vi "Adam_server_messages.vi"(1 "Filename":path) -> ()   [LabVIEW 2015]
panel:
  out "String":string
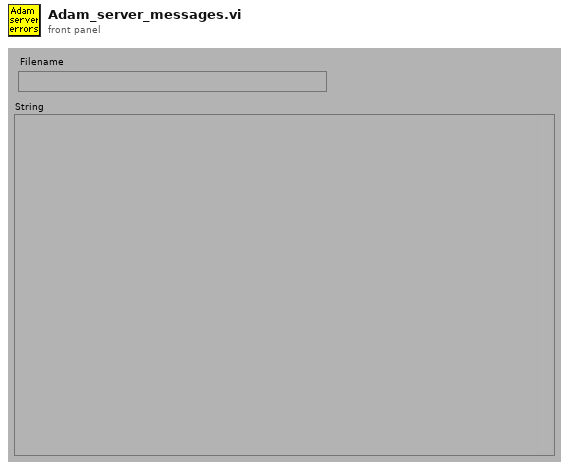
[diagram p1: front panel]
types:
  T1 = typedef "Ch_description_ADAM.ctl" = cluster{"Ch Name":string, "Type":T2, "Function":T3, "Ch State":T4, "Calibration type":T5, "A":dbl, "B":dbl, "C":dbl, "D":dbl, "Comments":string, "Address":T6, "String":string, "Duty":u16}
  T2 = typedef "Module_type_ADAM.ctl" = string
  T3 = typedef "Function_ADAM.ctl" = enum16{"Analogue Input", "Digital Input", "Event counter", "Event rate", "Analogue Output", "Digital Output", "Relay Output"}
  T4 = typedef "Channel_State.ctl" = enum16{"On", "Off", "Always On", "Always Off"}
  T5 = typedef "Calib_type_ADAM.ctl" = enum16{"Raw", "Bx + A", "Cx^2 + Bx + A", "Dx^3 + Cx^2 + Bx + A", "In Band", "Hi-Tec Q", "Hi-Tec M_dot", "Text"}
  T6 = typedef "Address.ctl" = cluster{"Main":i32, "Ch.":i32, "Sub":i32, "Port Name":string}
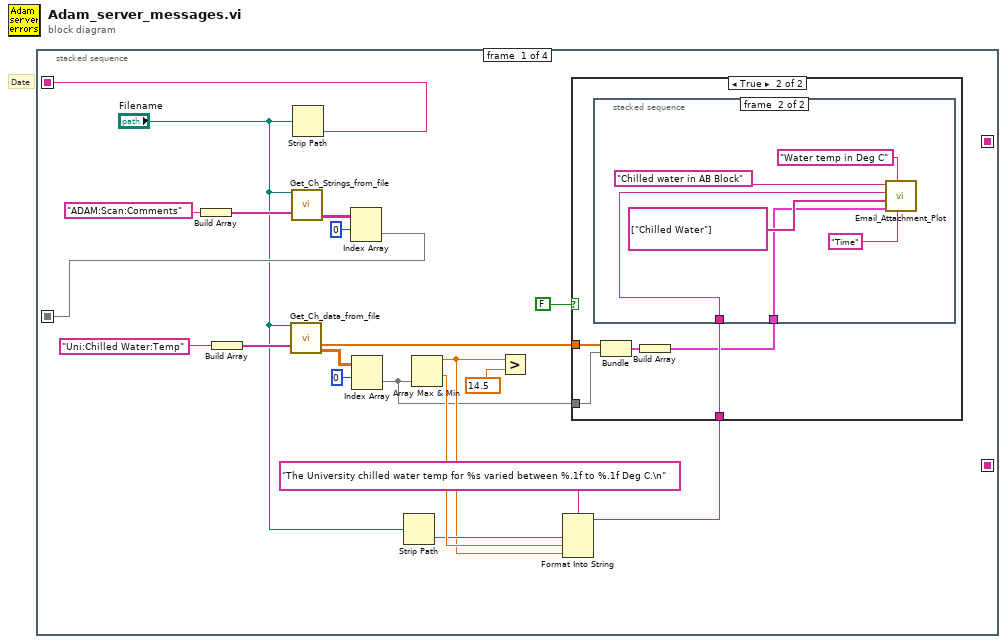
[diagram p0: block diagram]
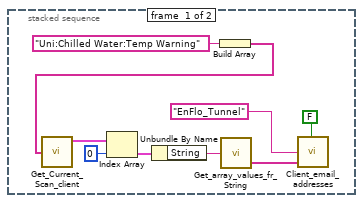
[diagram p3: hidden frame]
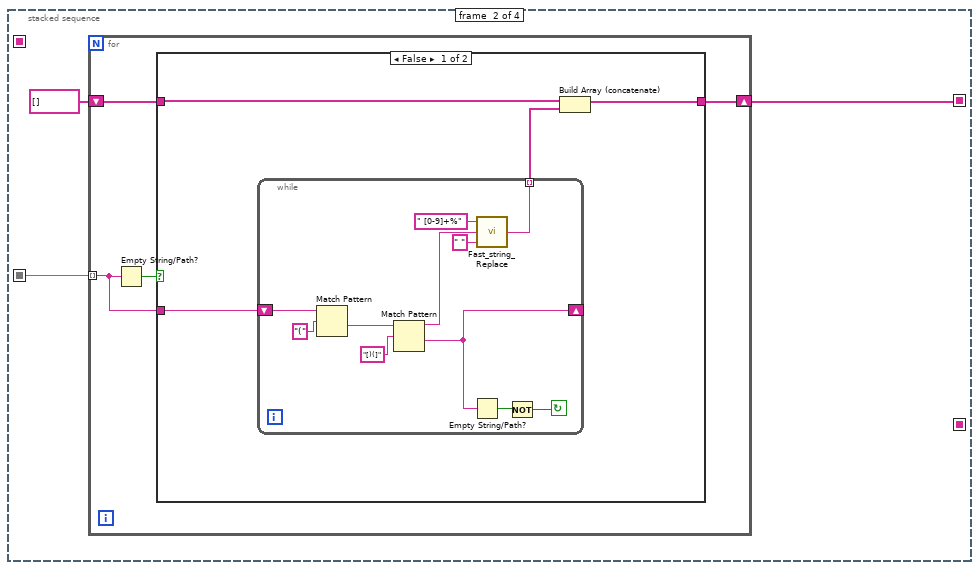
[diagram p4: hidden frame]
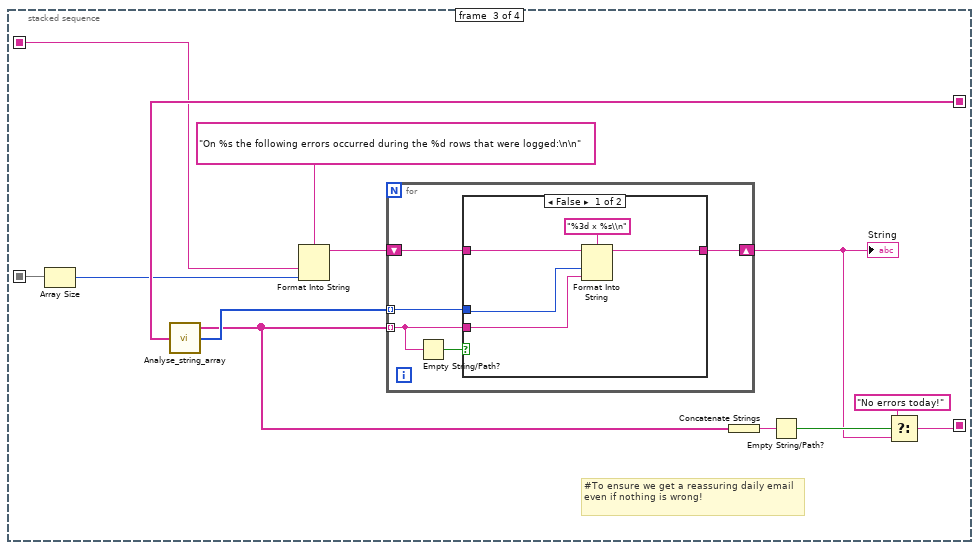
[diagram p6: hidden frame]
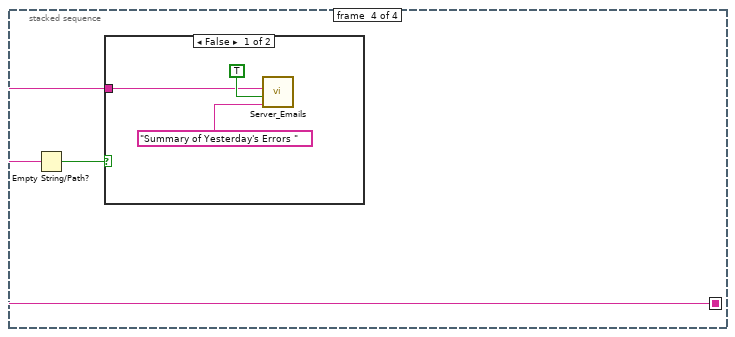
[diagram p8: hidden frame]
diagram:
  # "Date"
  n1 = stacked-sequence {
    seq-local: [w16 _ _ _] -> [_ w43 w73 _]
    seq-local: [_ w41 _ _] -> [_ _ w76 _]
    seq-local: [w15 _ _ _] -> [_ _ w64 _]
    seq-local: [_ _ w68 _] -> [_ _ _ w88]
    frame #0 {
      n2 = Build Array("ADAM:Scan:Comments") -> (w19:string[])
      n3 = Build Array("Uni:Chilled Water:Temp") -> (w3:string[])
      n4 = call "Get_Ch_data_from_file.vi"("Filename"="Filename", "Channel names"=w3) -> ("Times"=w4:dbl[], "Ch Data"=w7:dbl[][])  [unwired: 2 in, 10 out]
      n5 = call "Get_Ch_Strings_from_file.vi"("Filename"="Filename", "Channel names"=w19) -> ("Ch Data"=w17:string[][])  [unwired: 1 in, 12 out]
      n6 = Strip Path(path="Filename") -> (name=w15:string)  [unwired: 1 out]
      n7 = Index Array(array=w17, index (row)=0 ("Index")) -> (element=w16:string[])  [unwired: 1 in]
      n8 = Index Array(array=w7, index (row)=0 ("Index")) -> (element=w6:dbl[])  [unwired: 1 in]
      n9 = Strip Path(path="Filename") -> (name=w10:string)  [unwired: 1 out]
      n10 = Array Max & Min(array=w6) -> (max value=w9:dbl, min value=w11:dbl)  [unwired: 2 out]
      n11 = Greater?(x=w9, y=14.5 ("x")) -> ()  [unwired: 1 out]
      n12 = Format Into String(format string="The University chilled water temp for %s varied between %.1f to %.1f Deg C.\n" ("Format String"), w10, w11, w9) -> (resulting string=w5:string)  [unwired: 2 in, 1 out]
      n13 = case shown="True" FALSE {
        tunnel: w4 -> [_ w24]
        tunnel: w6 -> [_ w23]
        tunnel: w5 -> [_ w22]
        frame False {
        }
        frame True {
          n14 = Bundle("Times"=w24, "Ch Data"=w23) -> (w25:cluster{"Times":dbl[], "Ch Data":dbl[]})  [unwired: 1 out]
          n15 = Build Array(w25) -> (w21:cluster{"Times":dbl[], "Ch Data":dbl[]}[])
          n16 = stacked-sequence {
            tunnel: w22 -> [_ w36]
            tunnel: w21 -> [_ w35]
            frame #0 {
              n17 = Build Array("Uni:Chilled Water:Temp Warning") -> (w26:string[])
              n18 = call "Get_Current_Scan_client.vi"("ADAM Ch Names"=w26) -> ("Ch Description Array"=w34:T1[])  [unwired: 3 out]
              n19 = Index Array(array=w34, index=0) -> (element=w32:T1)
              n20 = Unbundle By Name(w32) -> ("String"=w31:string)
              n21 = call "Get_array_values_fr_String.vi"("String Value"=w31) -> ("String array"=w30:string[])  [unwired: 1 out]
              n22 = call "Client_email_addresses.vi"("Extra People to Email"=w30, "Client Name Contains"="EnFlo_Tunnel", "Contact All clients?"=FALSE) -> ()
            }
            frame #1 {
              n23 = call "Email_Attachment_Plot.vi"("X axis name"="Time", "Y axis name"="Water temp in Deg C", "XY Graph"=w35, "Series Names"=string[] ["Chilled Water"], "message"=w36, "subject ([No Subject])"="Chilled water in AB Block") -> ()  [unwired: 1 out]
            }
          }
        }
      }
    }
    frame #1 {
      n24 = for {
        shift-right: [w46] -> w41
        shift-left: string[] [] -> [w45]
        tunnel: w43 -> [w44] mode=indexing
        n25 = Empty String/Path?(string/path=w44) -> (empty?=w47:bool)
        n26 = case shown="False" w47 {
          tunnel: [w48 w63] -> w46
          tunnel: w45 -> [w49 w63]
          tunnel: w44 -> [w51 _]
          frame False {
            n27 = while {
              tunnel: [w53] -> w50 mode=indexing
              shift-left: w51 -> [w61]
              shift-right: [w58] -> _
              stop <- w56 continue-if-true
              n28 = Match Pattern(string=w61, regular expression="(") -> (after substring=w59:string)  [unwired: 4 out]
              n29 = Match Pattern(string=w59, regular expression="[)(]") -> (before substring=w55:string, after substring=w58:string)  [unwired: 3 out]
              n30 = Empty String/Path?(string/path=w58) -> (empty?=w57:bool)
              n31 = call "Fast_string_Replace.vi"("Replace match with:"=" ", "Input String"=w55, "regular expression"=" [0-9]+%") -> ("Output String"=w53:string)  [unwired: 2 out]
              n32 = Not(x=w57) -> (.not. x?=w56:bool)
            }
            n33 = Build Array (concatenate)(w49, w50) -> (w48:string[])
          }
          frame True {
          }
        }
      }
    }
    frame #2 {
      # "#To ensure we get a reassuring daily email even if nothing is wrong!"
      n34 = Array Size(array=w73) -> (size(s)=w72:i32)
      n35 = call "Analyse_string_array.vi"("String array"=w76) -> ("Unique strings"=w70:string[], "Frequency"=w75:i32[])  [unwired: 1 out]
      n36 = Format Into String(format string="On %s the following errors occurred during the %d rows that were logged:\n\n" ("Format String"), w64, w72) -> (resulting string=w71:string)  [unwired: 2 in, 1 out]
      n37 = for {
        tunnel: w70 -> [w78] mode=indexing
        tunnel: w75 -> [w81] mode=indexing
        shift-right: [w79] -> w66
        shift-left: w71 -> [w80]
        n38 = Empty String/Path?(string/path=w78) -> (empty?=w77:bool)
        n39 = case shown="False" w77 {
          tunnel: w81 -> [w82 _]
          tunnel: w80 -> [w86 w87]
          tunnel: [w85 w87] -> w79
          tunnel: w78 -> [w83 _]
          frame False {
            n40 = Format Into String(format string="%3d x %s\\n" ("Format String"), initial string=w86, w82, w83) -> (resulting string=w85:string)  [unwired: 1 in, 1 out]
          }
          frame True {
          }
        }
      }
      "String" <- w66
      n41 = Concatenate Strings(w70) -> (w69:string)
      n42 = Empty String/Path?(string/path=w69) -> (empty?=w67:bool)
      n43 = Select(t="No errors today!", s=w67, f=w66) -> (s? t:f=w68:string)
    }
    frame #3 {
      n44 = Empty String/Path?(string/path=w88) -> (empty?=w89:bool)
      n45 = case shown="False" w89 {
        tunnel: w88 -> [w90 _]
        frame False {
          n46 = call "Server_Emails.vi"("Message"=w90, "Contact All clients?"=TRUE, "Subject"="Summary of Yesterday's Errors ") -> ()  [unwired: 2 in, 3 out]
        }
        frame True {
        }
      }
    }
  }
